vi "HB_DisplayLCD.vi"(8 "error in (no error)":errorcluster, 10 "Display string":string, 11 "“HBDeviceRef_in":T1) -> (0 "error out":errorcluster, 3 "“HBDeviceRef_out":T1)   [LabVIEW 2016]
uses:
  <vilib>/Rock Robotics/WPI/SerialPort/WPI_SerialPortRef.ctl
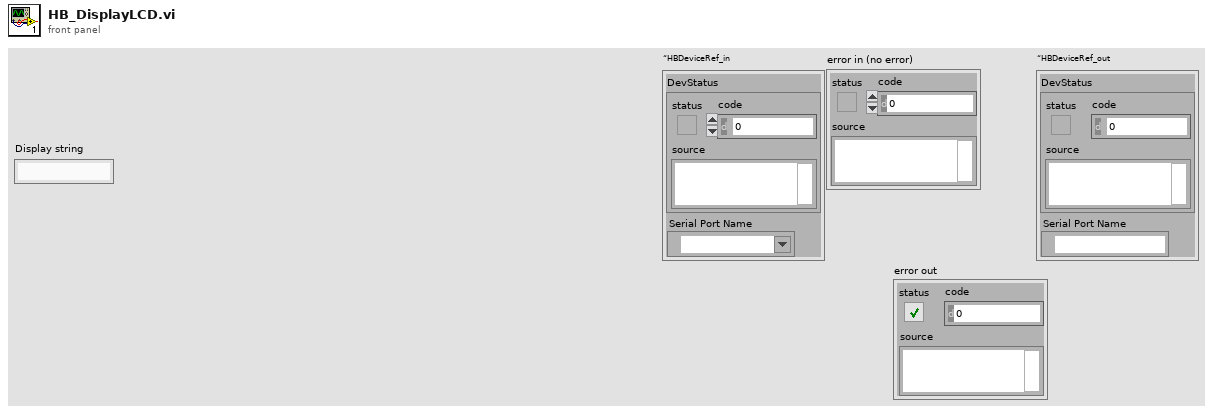
[diagram p1: front panel]
types:
  T1 = typedef "WPI_SerialPortRef.ctl" = cluster{"DevStatus":errorcluster, "Serial Port Name":refnum<visa-resource-name>}
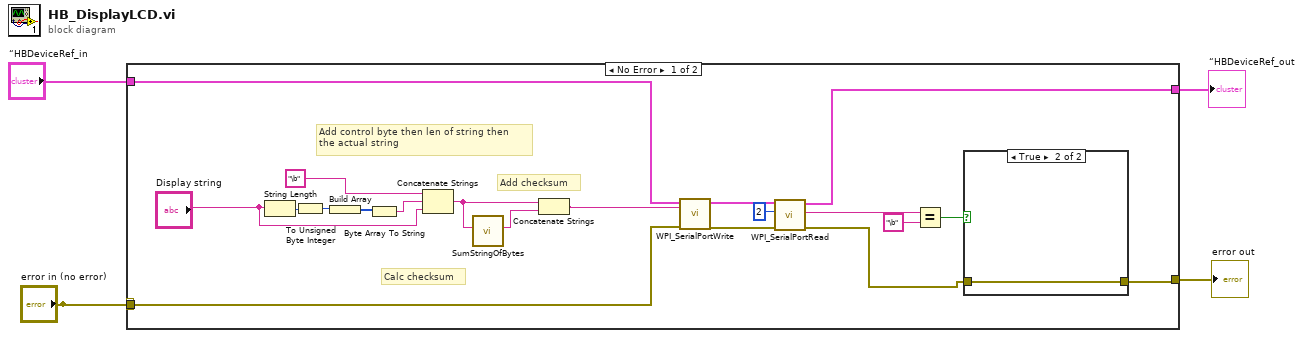
[diagram p0: block diagram]
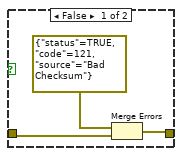
[diagram p2: hidden frame]
diagram:
  n1 = case shown="No Error" "error in (no error)" {
    selector: "error in (no error)" -> [_ w30]
    tunnel: "“HBDeviceRef_in" -> [w24 w29]
    tunnel: "error in (no error)" -> [w23 _]
    tunnel: [w20 w29] -> w3
    tunnel: [w14 w30] -> w2
    frame No Error {
      # "Calc checksum"
      # "Add checksum"
      # "Add control byte then len of string then \nthe actual string"
      n2 = String Length(string="Display string") -> (length=w13:i32)
      n3 = To Unsigned Byte Integer(number=w13) -> (unsigned 8bit integer=w10:u8)
      n4 = Build Array(w10) -> (w11:u8[])
      n5 = Byte Array To String(unsigned byte array=w11) -> (string=w12:string)
      n6 = Concatenate Strings("\b", w12, "Display string") -> (w8:string)
      n7 = call "SumStringOfBytes.vi"("String Of Bytes"=w8) -> ("SumAsString"=w7:string)  [unwired: 10 in]
      n8 = Concatenate Strings(w8, w7) -> (w6:string)
      n9 = call <vilib>:"WPI_SerialPortWrite.vi"("error in (no error)"=w23, "Buffer"=w6, "SerialPortRef"=w24) -> ("error out"=w21:errorcluster, "SerialPortRef"=w22:T1)  [unwired: 6 in, 1 out]
      n10 = call <vilib>:"WPI_SerialPortRead.vi"("error in (no error)"=w21, "Num Bytes to Read"=u32 2, "SerialPortRef"=w22) -> ("error out"=w15:errorcluster, "Buffer"=w18:string, "SerialPortRef"=w20:T1)  [unwired: 6 in]
      n11 = Equal?(x=w18, y="\b") -> (x = y?=w16:bool)
      n12 = case shown="True" w16 {
        tunnel: w15 -> [w26 w28]
        tunnel: [w27 w28] -> w14
        frame False {
          n13 = Merge Errors(errorcluster {"status"=TRUE, "code"=121, "source"="Bad Checksum"} ("error out"), w26) -> (w27:errorcluster)
        }
        frame True {
        }
      }
    }
    frame Error {
    }
  }
  "“HBDeviceRef_out" <- w3
  "error out" <- w2
